vi "Configure Trigger.vi"(8 "error in":errorcluster, 11 "DAQmx Base CFG in":refnum<class "DAQmx Base CFG.lvclass">) -> (0 "error out":errorcluster, 3 "DAQmx Base CFG out":refnum<class "DAQmx Base CFG.lvclass">)   [LabVIEW 2023, in "DAQmx Base CFG.lvclass"]
uses:
  DAQmx Base CFG.lvclass
  Configuration/Configuration JSON/Configuration JSON Base/CFG JSON.lvclass/CFG JSON.ctl
  ec36c310-6f2c-407d-a04f-30b9d6b93727.vi
  <vilib>/JDP Science/JSONtext/Find Item.vi
  <vilib>/JDP Science/JSONtext/Next JSON Value.vi
  <vilib>/JDP Science/JSONtext/String Subset.vi
  <vilib>/JDP Science/JSONtext/Parsing/Advance past next JSON Value (inlined COPY).vi
  <vilib>/JDP Science/JSONtext/Parsing/Advance past whitespace.vi
  <vilib>/JDP Science/JSONtext/Parsing/Advance past String.vi
  <vilib>/JDP Science/JSONtext/Parsing/Advance past Number.vi
  <vilib>/JDP Science/JSONtext/Parsing/Advance past Line Ending.vi
  <vilib>/JDP Science/JSONtext/Parsing/Parse Full Path or Item Name.vi
  <vilib>/JDP Science/JSONtext/Parsing/Advance past Array.vi
  <vilib>/JDP Science/JSONtext/Parsing/Advance past Object.vi
  <vilib>/JDP Science/JSONtext/support/Error Cluster From Code.vi
  <vilib>/JDP Science/JSONtext/Offset/Find Item Locations by Path.vi
  <vilib>/JDP Science/JSONtext/JSON text to Variant.vi
  <vilib>/Utility/error.llb/Error Cluster From Error Code.vi
  <vilib>/JDP Science/JSONtext/LVClass Serializer/JSONtext LVClass Serializer.lvclass
  <vilib>/ErrorRing/Error Ring.xnode
  DAQmx Base CFG.lvclass/DAQmx Base CFG.ctl
  Configuration/Configuration JSON/Configuration JSON Base/CFG JSON.lvclass
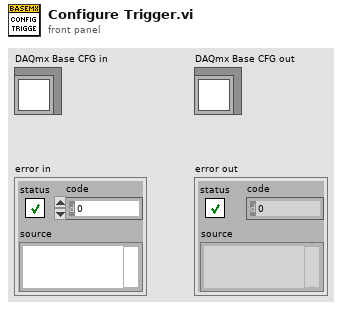
[diagram p1: front panel]
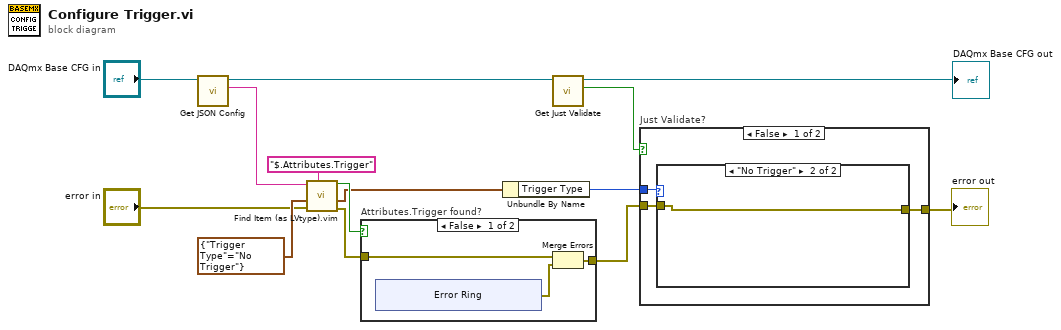
[diagram p0: block diagram]
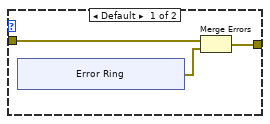
[diagram p2: hidden frame]
diagram:
  n1 = call "Get JSON Config.vi"("CFG Base in"="DAQmx Base CFG in") -> ("<JSON>Config>"=w14:string, "CFG Base out"=w1:refnum<class "DAQmx Base CFG.lvclass">)  [unwired: 9 in]
  n2 = call "Find Item (as LVtype).vim"("$Path or Item Name"="$.Attributes.Trigger", "error in (no error)"="error in", "Data Type and Default Value"=cluster{"Trigger Type":enum16{"No Trigger"}} {"Trigger Type"=enum."No Trigger"}, "JSON"=w14) -> ("error out"=w11:errorcluster, "Data"=w9:cluster{"Trigger Type":enum16{"No Trigger"}}, "Found"=w10:bool)  [unwired: 4 in, 1 out]
  n3 = case "Attributes.Trigger found?" shown="False" w10 {
    tunnel: w11 -> [w16 w23]
    tunnel: [w15 w23] -> w7
    frame False {
      n4 = xnode "Error Ring"() -> ("error out"=w17:errorcluster)
      n5 = Merge Errors(w16, w17) -> (w15:errorcluster)
    }
    frame True {
    }
  }
  n6 = Unbundle By Name(w9) -> ("Trigger Type"=w8:enum16{"No Trigger"})
  n7 = call "Get Just Validate.vi"("CFG JSON Base in"=w1) -> ("Just Validate"=w4:bool, "CFG JSON Base out"=→"DAQmx Base CFG out":refnum<class "DAQmx Base CFG.lvclass">)  [unwired: 9 in]
  n8 = case "Just Validate?" shown="False" w4 {
    tunnel: w8 -> [w26 _]
    tunnel: w7 -> [w25 w36]
    tunnel: [w24 w36] -> w6
    frame False {
      n9 = case shown="\"No Trigger\"" w26 {
        tunnel: w25 -> [w29 w35]
        tunnel: [w27 w35] -> w24
        frame Default {
          n10 = xnode "Error Ring"() -> ("error out"=w28:errorcluster)
          n11 = Merge Errors(w29, w28) -> (w27:errorcluster)
        }
        frame "No Trigger" {
        }
      }
    }
    frame True {
    }
  }
  "error out" <- w6
